vi "Load FPGA Interface.vi"(7 "Don't load":bool, 8 "error in (no error)":errorcluster) -> (0 "error out":errorcluster)   [LabVIEW 2026, in "TALOS.lvlib"]
doc: "This VI contains the list of all the AEgIS PCs names (machine names)."
uses:
  TALOS.lvlib
  Interfaces/FPGA Interface/FPGA Interface.lvclass
  Ancestor/Ancestor/Ancestor.lvclass/Ancestor.ctl
  Generate Error.vi
  FGV/Error Memory/Get Error Description.vi
  Get PC name.vi
  Ancestor/Ancestor/Read ID.vi
  Get Class Name.vi
  <vilib>/Utility/error.llb/Clear Errors.vi
  FGV/Error Memory/Error Memory Core.vi
  <vilib>/AdvancedString/Delimited String to 1D String Array.vi
  <vilib>/AdvancedString/Delimited String to 1D String Array (string).vi
  Circus Root Path.vi
  FGV/Error Memory/Error Crt Lvl checker.vi
  FGV/Error Memory/Error Memory Core.vi/40c8088d-b597-4017-91af-faa98e00292e.vi
  FGV/Error Memory/Error Memory Core.vi/d4a3ab98-063c-4e44-b43d-fbdcfe6c2be2.vi
  Global Memory.vi
  <vilib>/Utility/LVClass/Get LV Class Name.vi
  Is in Packed Library.vi
  TALOS Root path.vi
  Read CSV worksheet.vi
  Global Constants.vi
  <vilib>/Utility/error.llb/General Error Handler.vi
  <vilib>/Utility/config.llb/Open Config Data.vi
  <vilib>/Utility/config.llb/Get Section Names.vi
  <vilib>/Utility/config.llb/Get Key Names.vi
  <vilib>/Utility/config.llb/Read Key.vi
  <vilib>/Utility/config.llb/Read Key (String).vi
  <vilib>/Utility/config.llb/Close Config Data.vi
  Ancestor/Ancestor/Ancestor.lvclass
  <vilib>/Comparison/Equal/Equal Functor/Equal Functor.lvclass
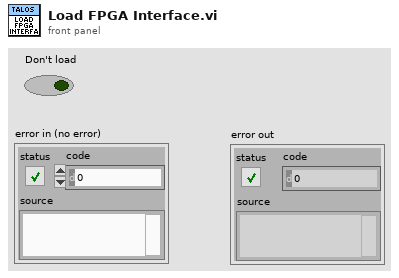
[diagram p1: front panel]
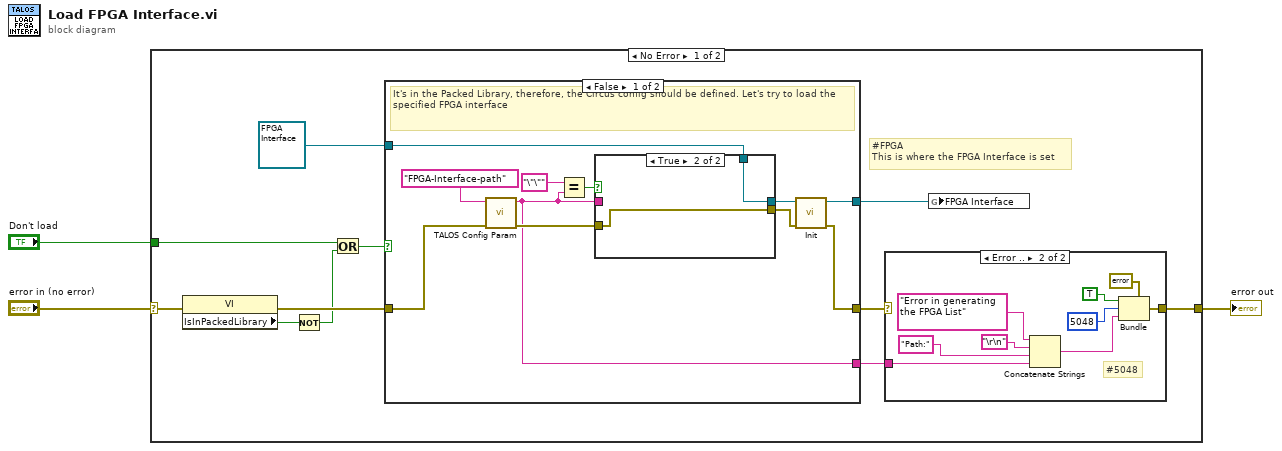
[diagram p0: block diagram]
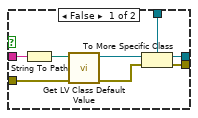
[diagram p2: hidden frame]
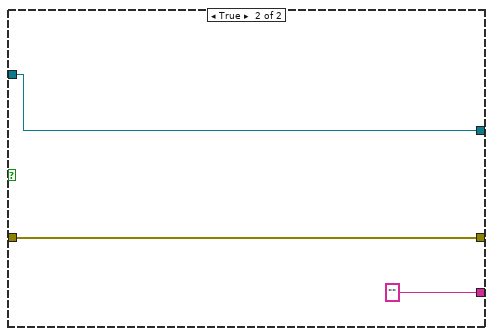
[diagram p3: hidden frame]
diagram:
  n1 = case shown="No Error" "error in (no error)" {
    selector: "error in (no error)" -> [w13 w49]
    tunnel: [w14 w49] -> w3
    tunnel: "Don't load" -> [w7 _]
    frame No Error {
      # "#FPGA\nThis is where the FPGA Interface is set"
      n2 = property class="VI"(error in=w13) -> (error out=w12:errorcluster, "IsInPackedLibrary"=w6:bool)  [unwired: 1 in, 1 out]
      n3 = Not(x=w6) -> (.not. x?=w5:bool)
      n4 = Or(x=w7, y=w5) -> (x .or. y?=w4:bool)
      n5 = case shown="False" w4 {
        tunnel: w12 -> [w21 w38]
        tunnel: [w23 w38] -> w11
        tunnel: [w24 w37] -> w10
        tunnel: refnum<class "FPGA Interface.lvclass"> refnum ("FPGA Interface") -> [w18 w37]
        tunnel: [w17 "" ("Value")] -> w8
        frame False {
          # "It's in the Packed Library, therefore, the Circus config should be defined. Let's try to load the specified FPGA interface"
          n6 = call "TALOS Config Param.vi"("error in (no error)"=w21, "Parameter Name"="FPGA-Interface-path") -> ("error out"=w20:errorcluster, "Output"=w17:string)  [unwired: 8 in]
          n7 = Equal?(x="\"\"", y=w17) -> (x = y?=w15:bool)
          n8 = case shown="True" w15 {
            tunnel: [w33 w35] -> w25
            tunnel: [w32 w34] -> w22
            tunnel: w20 -> [w29 w34]
            tunnel: w18 -> [w28 w35]
            tunnel: w17 -> [w26 _]
            frame False {
              n9 = String To Path(string=w26) -> (path=w27:path)
              n10 = call <vilib>:"Get LV Class Default Value.vi"("error in (no error)"=w29, "class path"=w27) -> ("error out"=w30:errorcluster, "object"=w31:refnum<class>)  [unwired: 8 in]
              n11 = To More Specific Class(target class=w28, reference=w31, error in=w30) -> (specific class reference=w33:refnum<class "FPGA Interface.lvclass">, error out=w32:errorcluster)
            }
            frame True {
            }
          }
          n12 = call-dynamic "Init.vi"("error in (no error)"=w22, "FPGA Interface in"=w25) -> ("error out"=w23:errorcluster, "FPGA Interface out"=w24:refnum<class "FPGA Interface.lvclass">)  [unwired: 8 in]
        }
        frame True {
        }
      }
      n13 = case shown="Error .." w11 {
        selector: w11 -> [w39 _]
        tunnel: [w39 w45] -> w14
        tunnel: w8 -> [_ w41]
        frame No Error {
        }
        frame Error {
          # "#5048"
          n14 = Concatenate Strings("Error in generating the FPGA List" ("source"), "\r\n", "Path:" ("string"), w41) -> (w40:string)
          n15 = Bundle(cluster=errorcluster {"status"=FALSE, "code"=0, "source"=""} ("error IO"), "status"=TRUE, "code"=5048, "source"=w40) -> (w45:errorcluster)
        }
      }
      n16 = global write "Global Memory.vi" "FPGA Interface"(w10) -> ()
    }
    frame Error {
    }
  }
  "error out" <- w3
